vi "PeriodicVisionKangaroo.vi"   [LabVIEW 2016]
uses:
  <vilib>/Rock Robotics/Network Tables/NT Write Number.vi
  <vilib>/Rock Robotics/Network Tables/NT Write String.vi
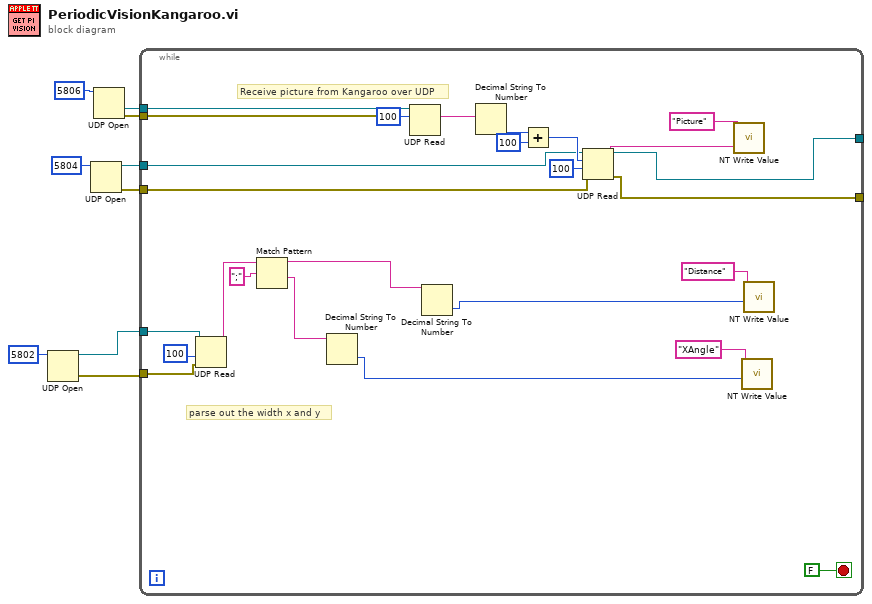
[diagram p0: block diagram]
diagram:
  n1 = UDP Open(11:u16 5802 ("port")) -> (port=w3:refnum<k16>, 0:w2:errorcluster)  [unwired: 4 in, 1 out]
  n2 = UDP Open(11:u16 5804 ("port")) -> (port=w7:refnum<k16>, 0:w8:errorcluster)  [unwired: 4 in, 1 out]
  n3 = UDP Open(11:u16 5806 ("port")) -> (port=w5:refnum<k16>, 0:w6:errorcluster)  [unwired: 4 in, 1 out]
  n4 = while {
    tunnel: w8 -> [w27]
    tunnel: w7 -> [w26]
    tunnel: w6 -> [w25]
    tunnel: w5 -> [w24]
    tunnel: [w22] -> _
    tunnel: [w21] -> _
    tunnel: w3 -> [w17]
    tunnel: w2 -> [w16]
    stop <- FALSE stop-if-true
    # "parse out the width x and y"
    # "Receive picture from Kangaroo over UDP"
    n5 = UDP Read(connection ID=w17, timeout ms (25000)=100, 8:w16) -> (data out=w18:string)  [unwired: 1 in, 4 out]
    n6 = Match Pattern(string=w18, regular expression=";") -> (before substring=w15:string, after substring=w14:string)  [unwired: 1 in, 2 out]
    n7 = Decimal String To Number(string=w14) -> (number=w10:i32)  [unwired: 2 in, 1 out]
    n8 = UDP Read(connection ID=w24, max size (548)=100, 8:w25) -> (data out=w34:string)  [unwired: 1 in, 4 out]
    n9 = Decimal String To Number(string=w15) -> (number=w13:i32)  [unwired: 2 in, 1 out]
    n10 = Decimal String To Number(string=w34) -> (number=w33:i32)  [unwired: 2 in, 1 out]
    n11 = Add(x=w33, y=100) -> (x+y=w31:i32)
    n12 = UDP Read(connection ID=w26, max size (548)=w31, timeout ms (25000)=100, 8:w27) -> (data out=w28:string, error out=w21:errorcluster, 3:w22:refnum<k16>)  [unwired: 2 out]
    n13 = call-poly <vilib>:"NT Write Value.vi"("String"=w28, "Name"="Picture") -> ()  [unwired: 9 in, 1 out]
    n14 = call-poly <vilib>:"NT Write Value.vi"("Numeric"=w10, "Name"="XAngle") -> ()  [unwired: 9 in, 1 out]
    n15 = call-poly <vilib>:"NT Write Value.vi"("Numeric"=w13, "Name"="Distance") -> ()  [unwired: 9 in, 1 out]
  }
